vi "Zadanie2.vi"() -> ()   [LabVIEW 2024]
panel:
  out "Out":i32
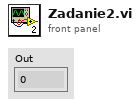
[diagram p1: front panel]
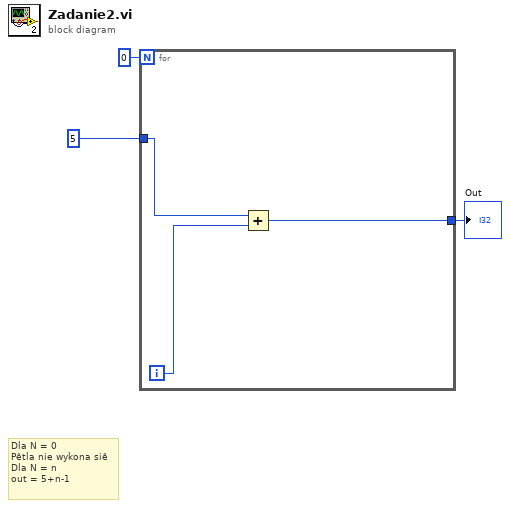
[diagram p0: block diagram]
diagram:
  # "Dla N = 0 \nPêtla nie wykona siê\nDla N = n\nout = 5+n-1"
  n1 = for {
    N: 0 -> [_]
    tunnel: 5 -> [w6]
    tunnel: [w4] -> w1
    i -> [w5]
    n2 = Add(x=w6, y=w5) -> (x+y=w4:i32)
  }
  "Out" <- w1
